vi "elapsed time example.vi"() -> ()   [LabVIEW 2013]
panel:
  out "Test Time":dbl
  out "error out":errorcluster
  in  "error in (no error)":errorcluster
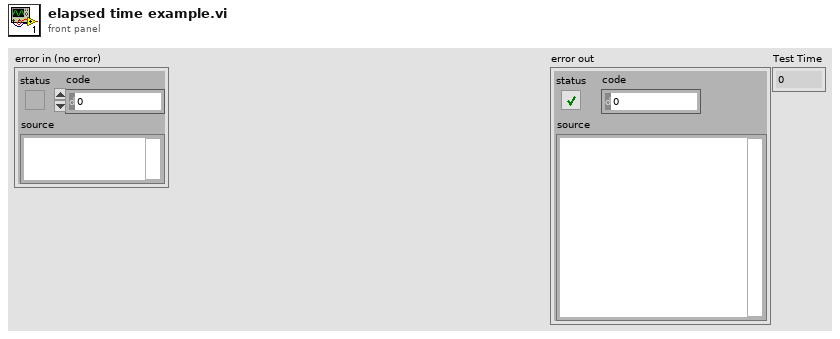
[diagram p1: front panel]
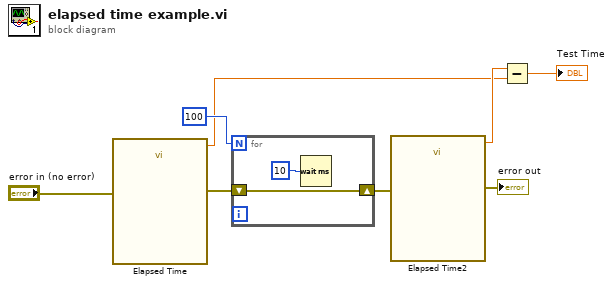
[diagram p0: block diagram]
diagram:
  n1 = call "Elapsed Time"("error in (no error)"="error in (no error)") -> ("Present (s)"=w2:dbl, "error out"=w5:errorcluster)  [unwired: 11 in, 6 out]
  n2 = for {
    N: 100 -> [_]
    shift-right: [w10] -> w6
    shift-left: w5 -> [w10]
    n3 = Wait (ms)(milliseconds to wait=u32 10) -> ()  [unwired: 1 out]
  }
  n4 = call "Elapsed Time2"("error in (no error)"=w6) -> ("Present (s)"=w3:dbl, "error out"=→"error out":errorcluster)  [unwired: 11 in, 6 out]
  n5 = Subtract(x=w3, y=w2) -> (x-y=→"Test Time":dbl)
